vi "Load Plot Grid.vi"() -> ()   [LabVIEW 2013]
uses:
  <vilib>/Utility/miscctls.llb/LV3DPointTypeDef.ctl
  Cube/Grid.lvclass/Grid.ctl
  <vilib>/Analysis/coordinate.llb/3D Coordinate Conversion (Scalar).vi
  <vilib>/Analysis/NI_AALPro.lvlib
  Cerebellum/Cerebellum.lvclass
  Cube/Grid.lvclass
panel:
  out "No Neurons":i32
  out "error out":errorcluster
  in  "stop":bool
  in  "Camera Position":cluster{"X":sgl, "Y":sgl, "Z":sgl}={"X"=0.0, "Y"=250.0, "Z"=100.0}
  out "3D Picture":refnum<vi>(3d-picture)
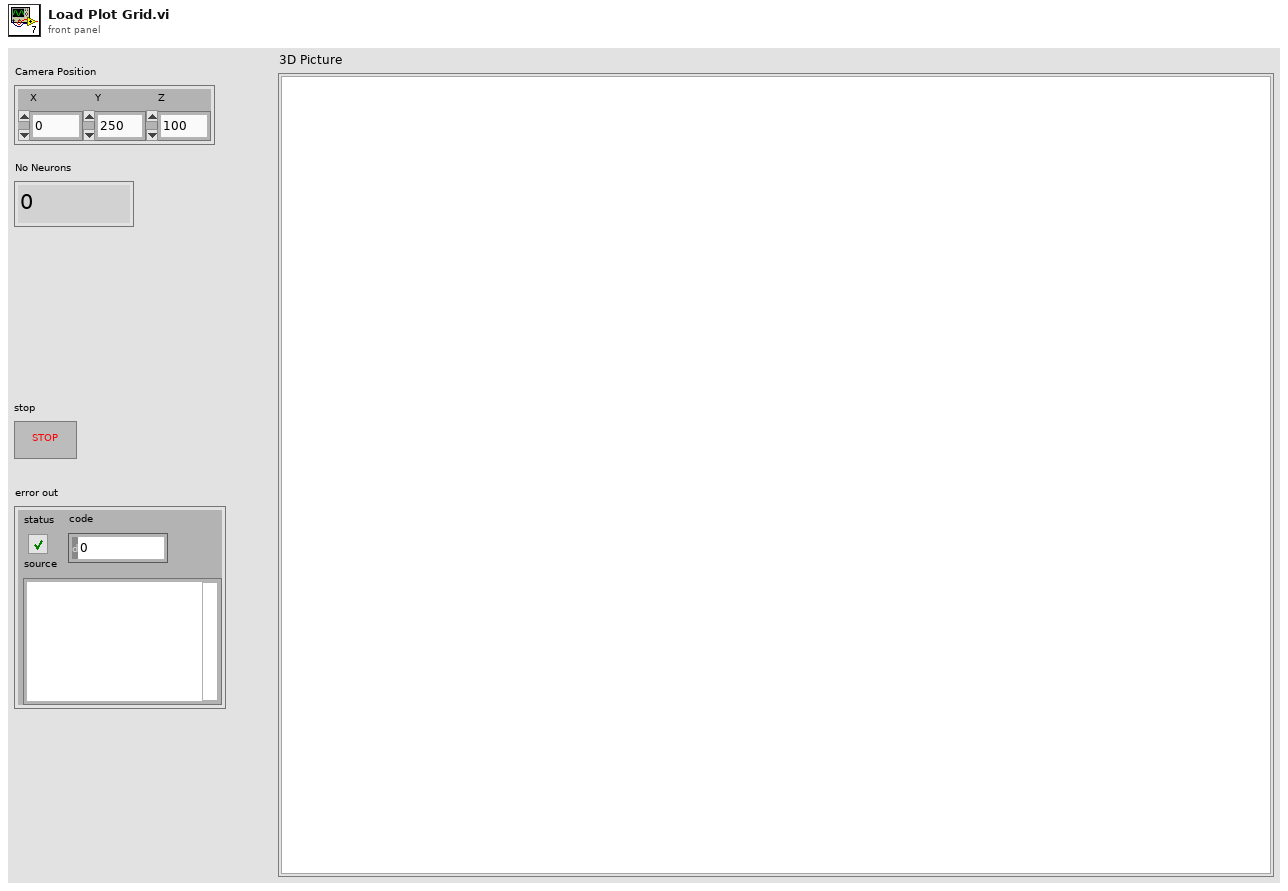
[diagram p1: front panel]
types:
  T1 = typedef "LV3DPointTypeDef.ctl" = cluster{"X":sgl, "Y":sgl, "Z":sgl}
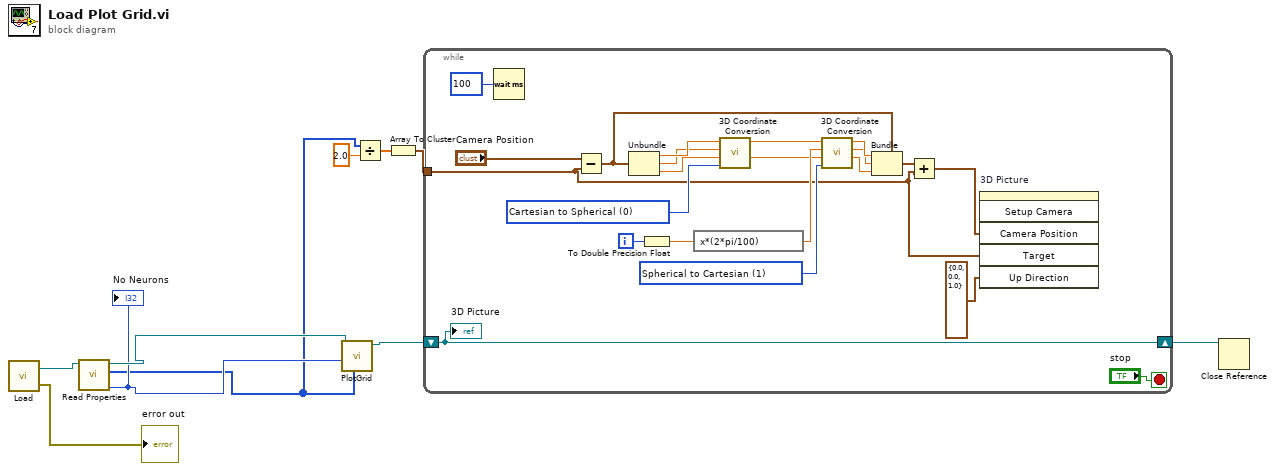
[diagram p0: block diagram]
diagram:
  n1 = call "Load.vi"() -> ("Grid out"=w7:refnum<class "Grid.lvclass">, "error out"=→"error out":errorcluster)  [unwired: 1 in]
  n2 = call "Read Properties.vi"("Grid in"=w7) -> ("No Neurons"=w5:i32, "Size(um)"=w2:u32[], "Grid out"=w6:refnum<class "Grid.lvclass">)  [unwired: 6 in, 2 out]
  "No Neurons" <- w5
  n3 = call "PlotGrid.vi"("Size (um)"=w2, "No Neurons"=w5, "Grid in"=w6) -> ("Scene Object Out"=w8:refnum<vi>)  [unwired: 8 in]
  n4 = Divide(x=w2, y=2.0 ("Numeric")) -> (x/y=w3:dbl[])
  n5 = Array To Cluster(array=w3) -> (cluster=w1:cluster{"[0]":dbl, "[1]":dbl, "[2]":dbl})
  n6 = while {
    shift-right: [w32] -> w10
    shift-left: w8 -> [w32]
    tunnel: w1 -> [w11]
    i -> [w27]
    stop <- "stop" stop-if-true
    w24 = u16 1 items=["Cartesian to Spherical", "Spherical to Cartesian", "Cartesian to Cylindrical", "Cylindrical to Cartesian", "Spherical to Cylindrical", "Cylindrical to Spherical"] ("conversion type")
    w28 = u16 0 items=["Cartesian to Spherical", "Spherical to Cartesian", "Cartesian to Cylindrical", "Cylindrical to Cartesian", "Spherical to Cylindrical", "Cylindrical to Spherical"] ("conversion type")
    n7 = Wait (ms)(milliseconds to wait=u32 100) -> ()  [unwired: 1 out]
    n8 = Subtract(x="Camera Position", y=w11) -> (x-y=w14:cluster{dbl, dbl, dbl})
    n9 = Unbundle(w14) -> (w31:dbl, w30:dbl, w29:dbl)
    n10 = To Double Precision Float(number=w27) -> (double precision float=w26:dbl)
    n11 = expression code="x*(2*pi/100)"(w26) -> (w17:dbl)
    n12 = call-poly <vilib>:"3D Coordinate Conversion.vi"("conversion type"=w28, "axis 3"=w29, "axis 2"=w30, "axis 1"=w31) -> ("axis 3 out"=w16:dbl, "axis 1 out"=w25:dbl)  [unwired: 4 in, 2 out]
    n13 = call-poly <vilib>:"3D Coordinate Conversion.vi"("conversion type"=w24, "axis 3"=w16, "axis 2"=w17, "axis 1"=w25) -> ("axis 3 out"=w21:dbl, "axis 2 out"=w22:dbl, "axis 1 out"=w23:dbl)  [unwired: 4 in, 1 out]
    n14 = Bundle(cluster=w14, w23, w22, w21) -> (w13:cluster{dbl, dbl, dbl})
    n15 = Add(x=w13, y=w11) -> (x+y=w12:cluster{dbl, dbl, dbl})
    n16 = invoke on="3D Picture" class="SceneGraphDisp (strict)" method="Setup Camera"("Camera Position"=w12, "Target"=w11, "Up Direction"=T1 {"X"=0.0, "Y"=0.0, "Z"=1.0}) -> ()  [unwired: 3 in, 6 out]
    "3D Picture" <- w32
  }
  n17 = Close Reference(reference=w10) -> ()  [unwired: 1 in, 1 out]
